vi "LinearSVR.vi"(8 "error in":errorcluster) -> (0 "error out":errorcluster, 3 "out":refnum<class "LinearSVR.lvclass">)   [LabVIEW 2020]
doc: "Linear Support Vector Regression.\n\n Similar to SVR with parameter kernel='linear', but implemented in terms of\n liblinear rather than libsvm, so it has more flexibility in the choice of\n penalties and loss functions and should scale better to large numbers of\n samples.\n\n This class supports both dense and sparse input.\n\n Read more in the :ref:`User Guide <svm_regression>`.\n\n .. versionadded:: 0.16\n\n Parameters\n ----------\n epsilon : float, default=0.0\n Epsilon parameter in the epsilon-insensitive loss function. Note\n that the value of this parameter depends on the scale of the target\n variable y. If unsure, set ``epsilon=0``.\n\n tol : float, default=1e-4\n Tolerance for stopping criteria.\n\n C : float, default=1.0\n Regularization parameter. The strength of the regularization is\n inversely proportional to C. Must be strictly positive.\n\n loss : {'epsilon_insensitive', 'squared_epsilon_insensitive'}, default='epsilon_insensitive'\n Specifies the loss function. The epsilon-insensitive loss\n (standard SVR) is the L1 loss, while the squared epsilon-insensitive\n loss ('squared_epsilon_insensitive') is the L2 loss.\n\n fit_intercept : bool, default=True\n Whether to calculate the intercept for this model. If set\n to false, no intercept will be used in calculations\n (i.e. data is expected to be already centered).\n\n intercept_scaling : float, default=1.\n When self.fit_intercept is True, instance vector x becomes\n [x, self.intercept_scaling],\n i.e. a \"synthetic\" feature with constant value equals to\n intercept_scaling is appended to the instance vector.\n The intercept becomes intercept_scaling * synthetic feature weight\n Note! the synthetic feature weight is subject to l1/l2 regularization\n as all other features.\n To lessen the effect of regularization on synthetic feature weight\n (and therefore on the intercept) intercept_scaling has to be increased.\n\n dual : bool, default=True\n Select the algorithm to either solve the dual or primal\n optimization problem. Prefer dual=False when n_samples > n_features.\n\n verbose : int, default=0\n Enable verbose output. Note that this setting takes advantage of a\n per-process runtime setting in liblinear that, if enabled, may not work\n properly in a multithreaded context.\n\n random_state : int, RandomState instance or None, default=None\n Controls the pseudo random number generation for shuffling the data.\n Pass an int for reproducible output across multiple function calls.\n See :term:`Glossary <random_state>`.\n\n max_iter : int, default=1000\n The maximum number of iterations to be run.\n\n Attributes\n ----------\n coef_ : ndarray of shape (n_features) if n_classes == 2 else (n_classes, n_features)\n Weights assigned to the features (coefficients in the primal\n problem).\n\n `coef_` is a readonly property derived from `raw_coef_` that\n follows the internal memory layout of liblinear.\n\n intercept_ : ndarray of shape (1) if n_classes == 2 else (n_classes)\n Constants in decision function.\n\n n_iter_ : int\n Maximum number of iterations run across all classes.\n\n \nAvailable methods:\nFit\nPredict\nScore\nGet Attributes\nGet Params\nSet Params"
uses:
  LinearSVR.lvclass
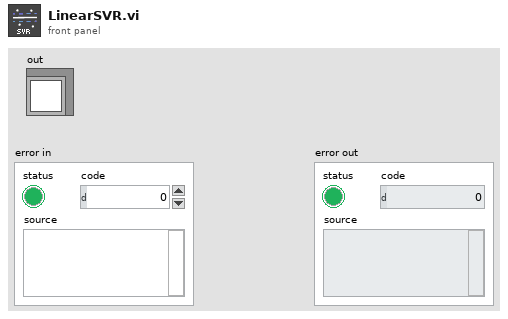
[diagram p1: front panel]
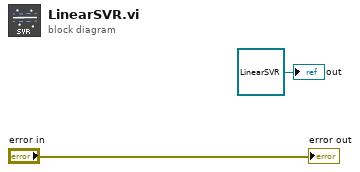
[diagram p0: block diagram]
diagram:
  "out" <- refnum<class "LinearSVR.lvclass"> refnum ("model")
  "error out" <- "error in"
